vi "Export to ProjFile Menu Entry.vi"(8 "error in (no error)":errorcluster, 11 "Menu Data in":refnum<class "Menu Data.lvclass">) -> (0 "error out":errorcluster, 2 "Menu Data":T1, 3 "Menu Data out":refnum<class "Menu Data.lvclass">)   [LabVIEW 2013, in "SET Project Data.lvlib" / "Menu Data.lvclass"]
uses:
  Menu Data.lvclass
  Types/ProjFile_Menu Data.ctl
  Menu Data.lvclass/Menu Data.ctl
  SET Project Data.lvlib
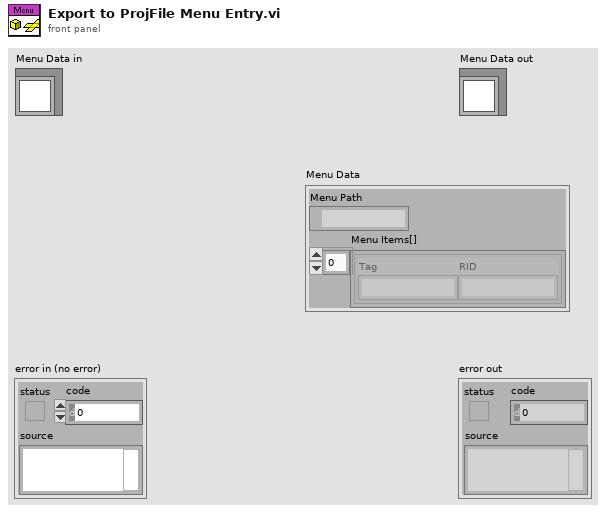
[diagram p1: front panel]
types:
  T1 = typedef "SET Project Data.lvlib/ProjFile_Menu Data.ctl" = cluster{"Menu Path":path, "Menu Items[]":cluster{"Tag":string, "RID":string}[]}
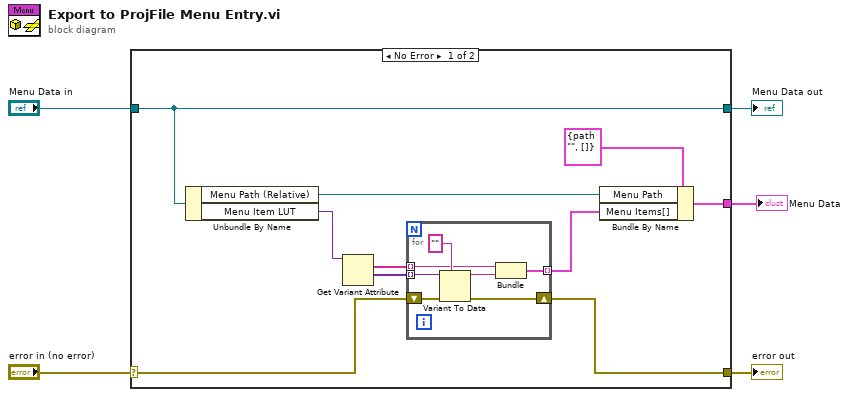
[diagram p0: block diagram]
diagram:
  n1 = case shown="No Error" "error in (no error)" {
    selector: "error in (no error)" -> [w7 w24]
    tunnel: [w6 w24] -> w4
    tunnel: [w14 w23] -> w2
    tunnel: "Menu Data in" -> [w14 w23]
    tunnel: [w8 _] -> w1
    frame No Error {
      n2 = Unbundle By Name(w14) -> ("Menu Path (Relative)"=w12:path, "Menu Item LUT"=w13:variant)
      n3 = Get Variant Attribute(Variant=w13) -> (names=w11:string[], values=w10:variant[])  [unwired: 3 in, 2 out]
      n4 = for {
        tunnel: w11 -> [w20] mode=indexing
        tunnel: w10 -> [w22] mode=indexing
        tunnel: [w18] -> w9 mode=indexing
        shift-right: [w16] -> w6
        shift-left: w7 -> [w17]
        n5 = Variant To Data(error in=w17, type="", Variant=w22) -> (data=w19:string, error out=w16:errorcluster)
        n6 = Bundle(w20, w19) -> (w18:cluster{string, string})  [unwired: 1 in]
      }
      n7 = Bundle By Name(cluster=T1 {"Menu Path"=path "", "Menu Items[]"=[]} ("Menu Data"), "Menu Path"=w12, "Menu Items[]"=w9) -> (w8:T1)
    }
    frame Error {
    }
  }
  "error out" <- w4
  "Menu Data out" <- w2
  "Menu Data" <- w1
